vi "FileWrite_CalConst.vi"(8 "error in":errorcluster, 10 "Calibration Constants":T1(array[cluster]) {"PSlope" format="%#.13f"; "NSlope" format="%#.13f"; "AvgSlope" format="%#.13f"; "Center" format="%#.13f"; "Offset" format="%#.13f"}, 11 "file path (use dialog)":path=path "") -> (0 "error out":errorcluster)   [LabVIEW 2015]
uses:
  <vilib>/Utility/file.llb/Write Delimited Spreadsheet (string).vi
panel:
  # "x1"
  # "x10"
  # "x100"
  # "x1000"
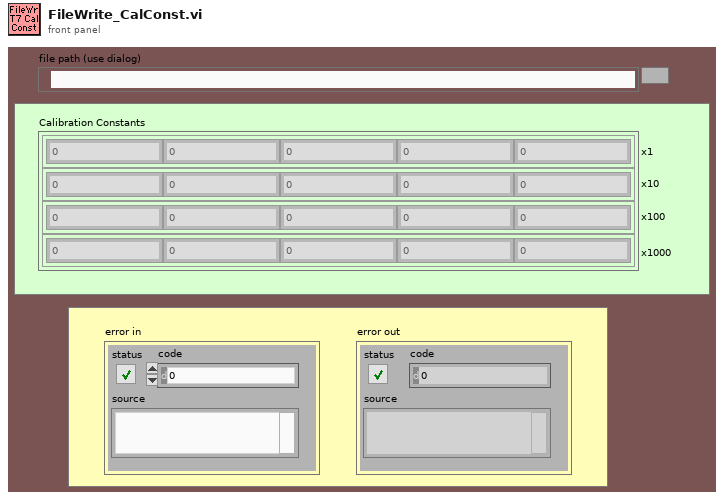
[diagram p1: front panel]
types:
  T1 = cluster{"PSlope":dbl, "NSlope":dbl, "AvgSlope":dbl, "Center":dbl, "Offset":dbl}[]
  T2 = enum16{"open", "replace", "create", "open or create", "replace or create", "replace or create with confirmation"}
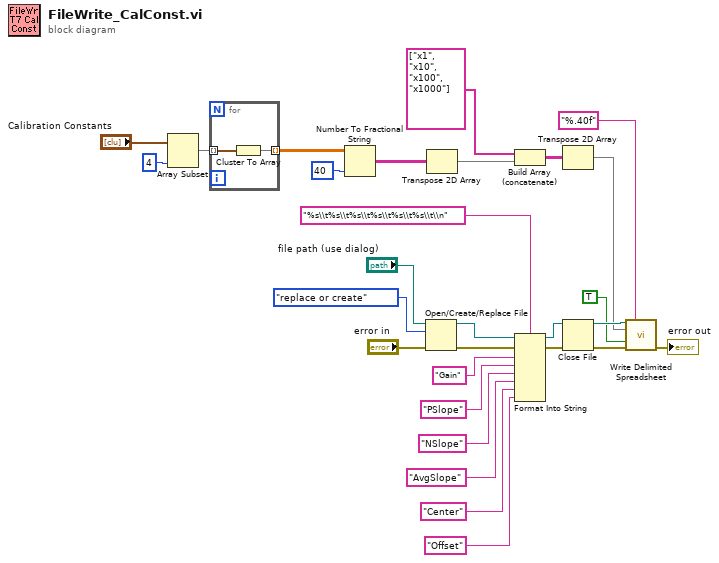
[diagram p0: block diagram]
diagram:
  n1 = Array Subset(array="Calibration Constants", length=4) -> (w28:T1)  [unwired: 1 in]
  n2 = for {
    tunnel: w28 -> [w31] mode=indexing
    tunnel: [w30] -> w14 mode=indexing
    n3 = Cluster To Array(cluster=w31) -> (array=w30:dbl[])
  }
  n4 = Number To Fractional String(number=w14, precision (6)=i16 40) -> (F-format string=w12:string[][])  [unwired: 2 in]
  n5 = Open/Create/Replace File(file path (use dialog)="file path (use dialog)", error in="error in", operation (0:open)=T2."replace or create") -> (refnum out=w23:refnum<file>, error out=w5:errorcluster)  [unwired: 3 in, 1 out]
  n6 = Transpose 2D Array(2D array=w12) -> (transposed array=w9:string[][])
  n7 = Build Array (concatenate)(string[] ["x1", "x10", "x100", "x1000"], w9) -> (w10:string[][])
  n8 = Format Into String(format string="%s\\t%s\\t%s\\t%s\\t%s\\t%s\\t\\n", initial string=w23, error in=w5, "Gain" ("input 1"), "PSlope", "NSlope", "AvgSlope", "Center", "Offset") -> (resulting string=w22:refnum<file>, error out=w4:errorcluster)
  n9 = Transpose 2D Array(2D array=w10) -> (transposed array=w8:string[][])
  n10 = Close File(refnum=w22, error in=w4) -> (path=w24:path, error out=w3:errorcluster)
  n11 = call-poly <vilib>:"Write Delimited Spreadsheet.vi"("file path (dialog if empty)"=w24, "format (%s)"="%.40f" ("format (%.3f)"), "2D data"=w8, "append to file? (F)"=TRUE, "error in (no error)"=w3) -> ("error out"=→"error out":errorcluster)  [unwired: 9 in, 1 out]
